vi "TranslatorBooster Search Tokens.vi"(10 "search tokens":string[](array[string]), 11 "input string":string) -> (0 "offset past token":i32, 1 "found token index":i32, 2 "output token":string, 3 "input string":string, 4 "actual token":string, 5 "token found?":bool)   [LabVIEW 2014, in "Complex Numbers.lvlib"]
uses:
  <vilib>/Aledyne-TSXperts/Arduino Compatible Compiler for LabVIEW/addons/Complex Numbers/Complex Numbers.lvlib
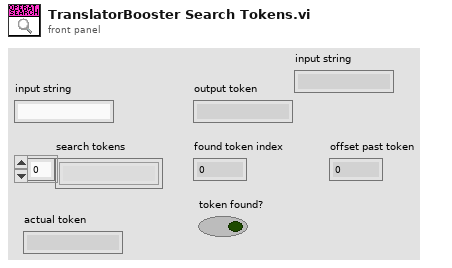
[diagram p1: front panel]
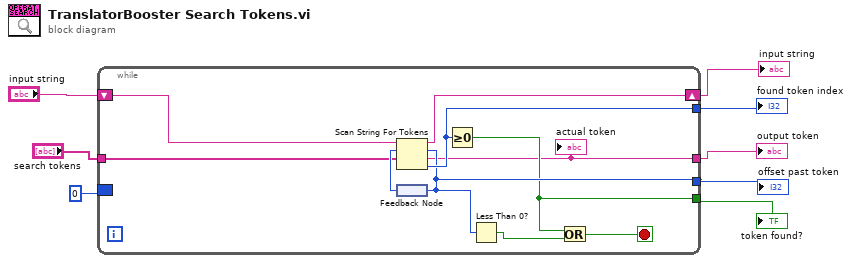
[diagram p0: block diagram]
diagram:
  n1 = while {
    border: 0 ("offset past token") -> [_]
    tunnel: [w15] -> w3
    tunnel: [w14] -> w2
    shift-right: [w12] -> w1
    shift-left: "input string" -> [w13]
    tunnel: [w11] -> w4
    tunnel: [w10] -> w7
    tunnel: "search tokens" -> [w9]
    stop <- w16 stop-if-true
    n2 = feedback #1() -> (w18:i32)
    n3 = Scan String For Tokens(7:w9, 8:w18, 9:w13) -> (0:w15:i32, 1:w10:string, 2:w14:i32, 3:w12:string)  [unwired: 3 in]
    "actual token" <- w10
    n4 = feedback-in #1(w14) -> ()
    n5 = Greater Or Equal To 0?(x=w15) -> (x >= 0?=w11:bool)
    n6 = Less Than 0?(x=w14) -> (x < 0?=w17:bool)
    n7 = Or(x=w11, y=w17) -> (x .or. y?=w16:bool)
  }
  "output token" <- w7
  "token found?" <- w4
  "found token index" <- w3
  "offset past token" <- w2
  "input string" <- w1
